vi "Process State(Close).vi"(0 "Process In":refnum<class "Process.lvclass">, 11 "Error In":errorcluster) -> (4 "Process Out":refnum<class "Process.lvclass">, 10 "Close?":bool, 15 "Error Out":errorcluster)   [LabVIEW 2023, in "Process.lvclass"]
doc: "Method encapsulating Close state of process."
uses:
  Process.lvclass
  Interfaces/ICanCommunicate/Message.ctl
  Process.lvclass/Process.ctl
  Interfaces/ICanCommunicate/ICanCommunicate.lvclass
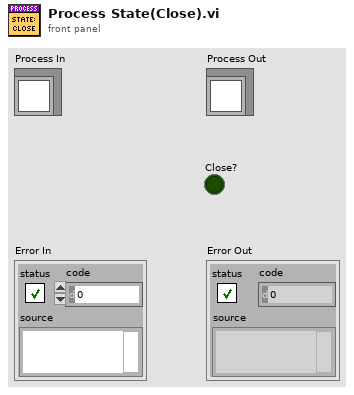
[diagram p1: front panel]
types:
  T1 = typedef "ICanCommunicate.lvclass/Message.ctl" = cluster{"Sender Name":string, "Recipent Name":string, "Command":string, "Data":variant, "Signature":string}
  T2 = typedef "ICanCommunicate.lvclass/ProcessSyncQueue.ctl" = refnum<queue>
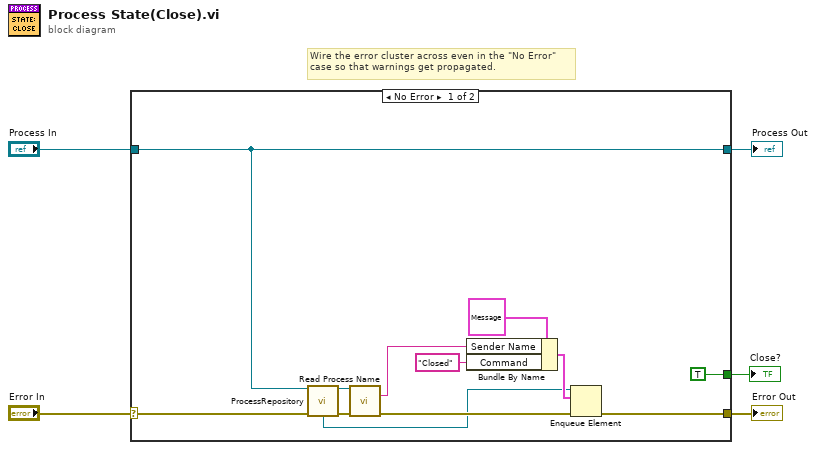
[diagram p0: block diagram]
diagram:
  # "Wire the error cluster across even in the \"No Error\"\ncase so that warnings get propagated."
  n1 = case shown="No Error" "Error In" {
    selector: "Error In" -> [w9 w19]
    tunnel: [w8 w19] -> w4
    tunnel: [w7 w18] -> w2
    tunnel: "Process In" -> [w7 w18]
    tunnel: [TRUE _] -> w1
    frame No Error {
      n2 = call-dynamic "ProcessRepository.vi"("Process In"=w7, "Error In"=w9) -> ("Process Out"=w16:refnum<class "Process.lvclass">, "ProcessSyncQueue"=w11:T2, "Error Out"=w10:errorcluster)  [unwired: 7 in, 4 out]
      n3 = call "Read Process Name.vi"("Process In"=w16, "Error In"=w10) -> ("Process Name"=w17:string, "Error Out"=w15:errorcluster)  [unwired: 11 in, 1 out]
      n4 = Bundle By Name(cluster=T1 {"Sender Name"="", "Recipent Name"="", "Command"="", "Data"=variant, "Signature"=""} ("element"), "Sender Name"=w17, "Command"="Closed") -> (w13:T1)
      n5 = Enqueue Element(queue=w11, element=w13, error in (no error)=w15) -> (error out=w8:errorcluster)  [unwired: 1 in, 2 out]
    }
    frame Error {
    }
  }
  "Error Out" <- w4
  "Process Out" <- w2
  "Close?" <- w1
